vi "Draw_Labels.vi"(7 "max value":dbl, 9 "last two points":cluster{dbl, dbl}[](array[cluster]), 10 "labels":cluster{"start":string, "end":string}[](array[cluster])=[{"start"="G3", "end"="A5"}, {"start"="0", "end"="10"}], 11 "picture in":picture) -> (3 "picture out":picture)   [LabVIEW 2022 SP3]
uses:
  Perspective_Globals.vi
panel:
  in  "[user-specified font]":T1={"Font Name:"="Arial", "Size"=12, "Strikeout?"=FALSE, "Italic?"=FALSE, "Underline?"=FALSE, "Outline?"=FALSE, "Shadow?"=FALSE, "Bold?"=FALSE}
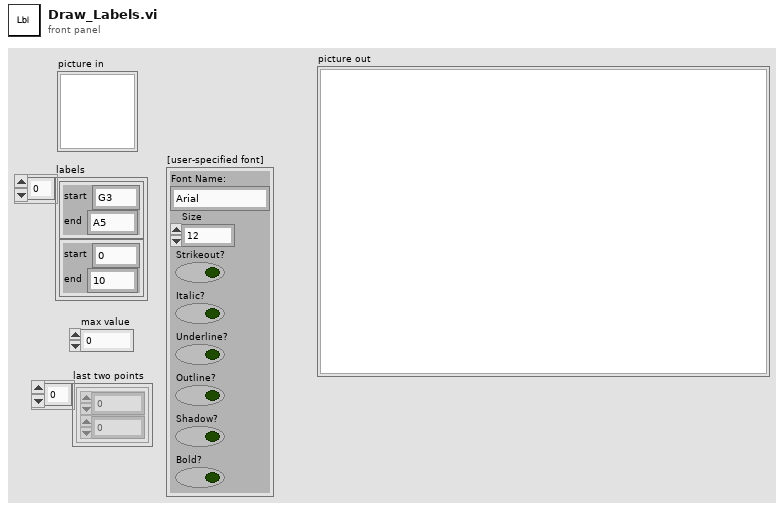
[diagram p1: front panel]
types:
  T1 = cluster{"Font Name:":string, "Size":i16, "Strikeout?":bool, "Italic?":bool, "Underline?":bool, "Outline?":bool, "Shadow?":bool, "Bold?":bool}
  T2 = enum16{"User-specified Font", "Application Font", "System Font", "Dialog Font"}
  T3 = cluster{"left":i16, "top":i16, "right":i16, "bottom":i16}
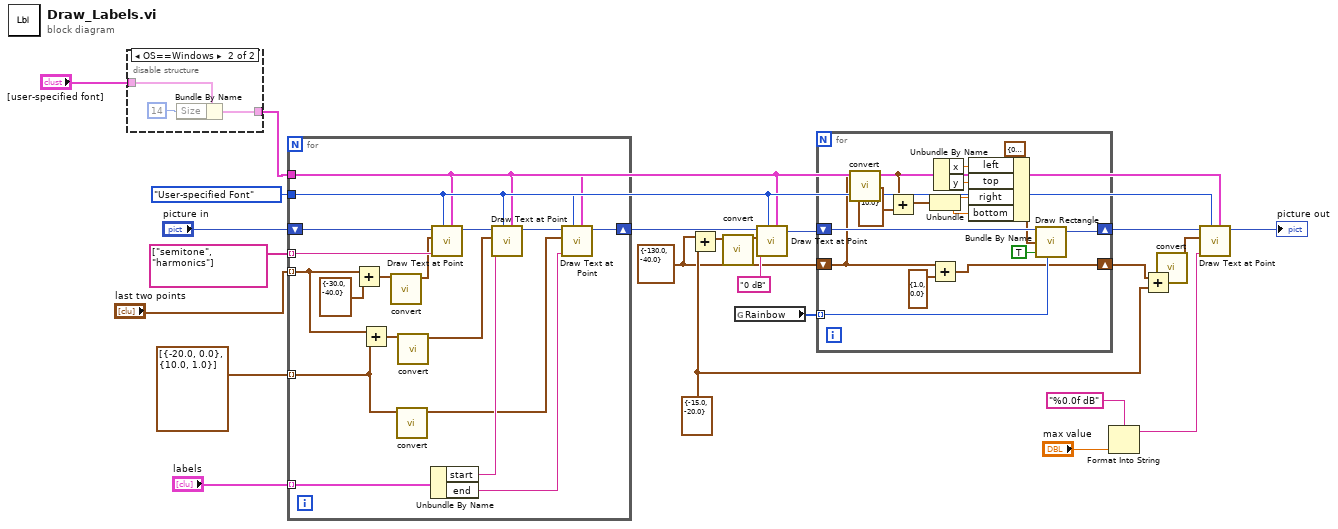
[diagram p0: block diagram]
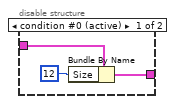
[diagram p2: hidden frame]
diagram:
  w5 = cluster{dbl, dbl} {-15.0, -20.0} ("y")
  w3 = T2."User-specified Font" ("desired font(Application)")
  w4 = cluster{dbl, dbl} {-130.0, -40.0} ("y")
  n1 = disable-structure shown="OS==Windows" {
    disable-tunnel: "[user-specified font]" -> [w27 w30]
    disable-tunnel: [w26 w29] -> w1
    frame condition #0 (active) {
      n2 = Bundle By Name(cluster=w27, "Size"=i16 12) -> (w26:T1)
    }
    frame condition #1 {
      n3 = Bundle By Name(cluster=w30, "Size"=i16 14) -> (w29:T1)
    }
  }
  n4 = for {
    shift-right: [w40] -> w7
    shift-left: "picture in" -> [w48]
    tunnel: string[] ["semitone", "harmonics"] -> [w47] mode=indexing
    tunnel: "last two points" -> [w36] mode=indexing
    tunnel: cluster{dbl, dbl}[] [{-20.0, 0.0}, {10.0, 1.0}] -> [w34] mode=indexing
    tunnel: "labels" -> [w33] mode=indexing
    tunnel: w1 -> [w32]
    tunnel: w3 -> [w31]
    n5 = Add(x=w36, y=cluster{dbl, dbl} {-30.0, -40.0}) -> (x+y=w44:cluster{dbl, dbl})
    n6 = Add(x=w36, y=w34) -> (x+y=w43:cluster{dbl, dbl})
    n7 = call "convert.vi"("point"=w44) -> ("scaled"=w45:cluster{"x":dbl, "y":dbl})  [unwired: 10 in]
    n8 = call "convert.vi"("point"=w34) -> ("scaled"=w35:cluster{"x":dbl, "y":dbl})  [unwired: 10 in]
    n9 = call "convert.vi"("point"=w43) -> ("scaled"=w39:cluster{"x":dbl, "y":dbl})  [unwired: 10 in]
    n10 = Unbundle By Name(w33) -> ("start"=w38:string, "end"=w37:string)
    n11 = call <vilib>:"Draw Text at Point.vi"("[user-specified font]"=w32, "desired font(Application)"=w31, "text"=w47, "origin"=w45, "picture"=w48) -> ("new picture"=w42:picture)  [unwired: 5 in, 1 out]
    n12 = call <vilib>:"Draw Text at Point.vi"("[user-specified font]"=w32, "desired font(Application)"=w31, "text"=w38, "origin"=w39, "picture"=w42) -> ("new picture"=w41:picture)  [unwired: 5 in, 1 out]
    n13 = call <vilib>:"Draw Text at Point.vi"("[user-specified font]"=w32, "desired font(Application)"=w31, "text"=w37, "origin"=w35, "picture"=w41) -> ("new picture"=w40:picture)  [unwired: 5 in, 1 out]
  }
  n14 = Add(x=w4, y=w5) -> (x+y=w10:cluster{dbl, dbl})
  n15 = call "convert.vi"("point"=w10) -> ("scaled"=w9:cluster{"x":dbl, "y":dbl})  [unwired: 10 in]
  n16 = global read "Perspective_Globals.vi" "Rainbow"() -> (w19:u32[])
  n17 = call <vilib>:"Draw Text at Point.vi"("[user-specified font]"=w1, "desired font(Application)"=w3, "text"="0 dB", "origin"=w9, "picture"=w7) -> ("new picture"=w6:picture)  [unwired: 5 in, 1 out]
  n18 = for {
    shift-right: [w63] -> w18
    shift-left: w6 -> [w64]
    tunnel: w19 -> [w62] mode=indexing
    shift-right: [w50] -> w12
    shift-left: w4 -> [w51]
    n19 = call "convert.vi"("point"=w51) -> ("scaled"=w56:cluster{"x":dbl, "y":dbl})  [unwired: 10 in]
    n20 = Add(x=w56, y=cluster{dbl, dbl} {1.0, 10.0}) -> (x+y=w54:cluster{dbl, dbl})
    n21 = Unbundle(w54) -> (w52:dbl, w53:dbl)
    n22 = Add(x=w51, y=cluster{dbl, dbl} {1.0, 0.0}) -> (x+y=w50:cluster{dbl, dbl})
    n23 = Unbundle By Name(w56) -> ("x"=w58:dbl, "y"=w57:dbl)
    n24 = Bundle By Name(cluster=T3 {"left"=0, "top"=0, "right"=0, "bottom"=0} ("rect"), "left"=w58, "top"=w57, "right"=w52, "bottom"=w53) -> (w59:T3)
    n25 = call <vilib>:"Draw Rectangle.vi"("picture"=w64, "rect"=w59, "fill?(F)"=TRUE, "color(black)"=w62) -> ("new picture"=w63:picture)  [unwired: 5 in]
  }
  n26 = Format Into String(format string="%0.0f dB", "max value") -> (resulting string=w14:string)  [unwired: 2 in, 1 out]
  n27 = Add(x=w12, y=w5) -> (x+y=w11:cluster{dbl, dbl})
  n28 = call "convert.vi"("point"=w11) -> ("scaled"=w13:cluster{"x":dbl, "y":dbl})  [unwired: 10 in]
  n29 = call <vilib>:"Draw Text at Point.vi"("[user-specified font]"=w1, "desired font(Application)"=w3, "text"=w14, "origin"=w13, "picture"=w18) -> ("new picture"=→"picture out":picture)  [unwired: 5 in, 1 out]
